vi "Read waveplate calibration file.vi"(8 "error in (no error)":errorcluster, 11 "file path (dialog if empty)":path) -> (0 "error out":errorcluster, 3 "Calibration array":cluster{"String":string, dbl}[](array[cluster]))   [LabVIEW 2013]
uses:
  <vilib>/Utility/file.llb/Read From Spreadsheet File (string).vi
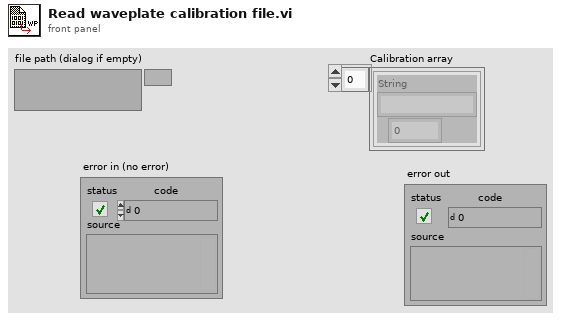
[diagram p1: front panel]
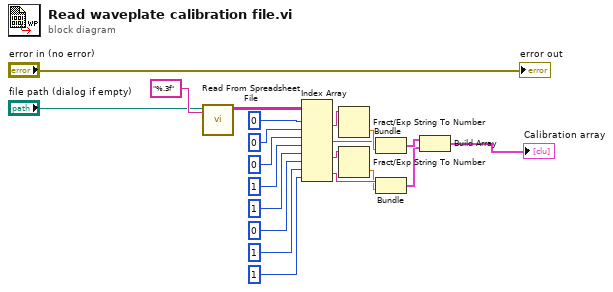
[diagram p0: block diagram]
diagram:
  n1 = call-poly <vilib>:"Read From Spreadsheet File.vi"("format (%s)"="%.3f" ("format (%.3f)"), "file path (dialog if empty)"="file path (dialog if empty)") -> ("all rows"=w11:string[][])  [unwired: 5 in, 4 out]
  n2 = Index Array(array=w11, index (row) #1=0 ("index"), index (col) #1=0 ("disabled index (col)"), index (row) #2=0 ("index"), index (col) #2=1 ("disabled index (col)"), index (row) #3=1 ("index (row)"), index (col) #3=0 ("disabled index (col)"), index (row) #4=1 ("index (row)"), index (col) #4=1 ("disabled index (col)")) -> (element #1=w12:string, element #2=w13:string, element #3=w20:string, element #4=w21:string)
  n3 = Fract/Exp String To Number(string=w12) -> (number=w14:dbl)  [unwired: 3 in, 1 out]
  n4 = Fract/Exp String To Number(string=w20) -> (number=w19:dbl)  [unwired: 3 in, 1 out]
  n5 = Bundle("String"=w13, w14) -> (w3:cluster{"String":string, dbl})  [unwired: 1 in]
  n6 = Bundle("String"=w21, w19) -> (w2:cluster{"String":string, dbl})  [unwired: 1 in]
  n7 = Build Array(w3, w2) -> (→"Calibration array":cluster{"String":string, dbl}[])
  "error out" <- "error in (no error)"
